vi "Request Parse.vi"(11 "WSGI Request":T2) -> (3 "Request":T1)   [LabVIEW 2021, in "HttpServer.lvlib"]
uses:
  HttpServer.lvlib
  TypeDefs/WSGI.ctl
  TypeDefs/Request.ctl
  <vilib>/Utility/miscctls.llb/LVMapReplaceAction.ctl
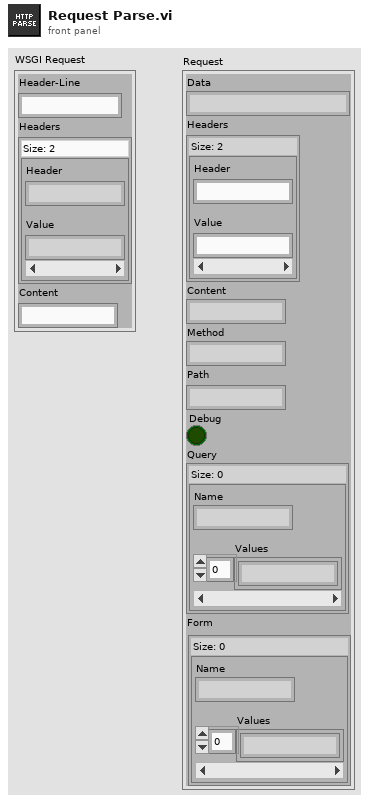
[diagram p1: front panel]
types:
  T1 = typedef "HttpServer.lvlib/Request.ctl" = cluster{"Data":string, "Headers":map{string, string}, "Content":string, "Method":string, "Path":string, "Debug":bool, "Query":map{string, string[]}, "Form":map{string, string[]}}
  T2 = typedef "HttpServer.lvlib/WSGI.ctl" = cluster{"Header-Line":string, "Headers":map{string, string}, "Content":string}
  T3 = typedef "LVMapReplaceAction.ctl" = enum32{"Modify Entry only if found", "Add or Modify Entry", "Delete Entry"}
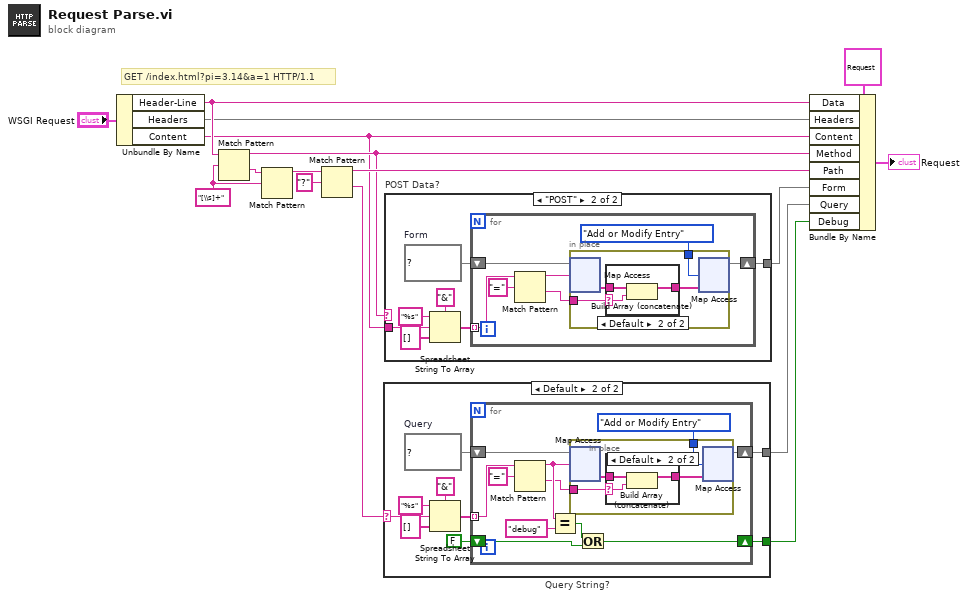
[diagram p0: block diagram]
diagram:
  w14 = "[\\s]+" ("regular expression")
  # "GET /index.html?pi=3.14&a=1 HTTP/1.1"
  n1 = Unbundle By Name("WSGI Request") -> ("Header-Line"=w11:string, "Headers"=w3:map{string, string}, "Content"=w2:string)
  n2 = Match Pattern(string=w11, regular expression=w14) -> (before substring=w4:string, after substring=w15:string)  [unwired: 1 in, 2 out]
  n3 = Match Pattern(string=w15, regular expression=w14) -> (before substring=w13:string)  [unwired: 1 in, 3 out]
  n4 = Match Pattern(string=w13, regular expression="?") -> (before substring=w10:string, after substring=w8:string)  [unwired: 1 in, 2 out]
  n5 = case "Query String?" shown="Default" w8 {
    selector: w8 -> [_ w22]
    tunnel: [_ w18] -> w6
    tunnel: [_ w17] -> w5
    frame "" {
    }
    frame Default {
      w20 = map{string, string[]} {}  # Query
      n6 = Spreadsheet String To Array(delimiter (Tab)="&", format string="%s", spreadsheet string=w22, array type (2D Dbl)=string[] []) -> (array=w21:string[])
      n7 = for {
        tunnel: w21 -> [w36] mode=indexing
        shift-right: [w27] -> w17
        shift-left: w20 -> [w30]
        shift-right: [w35] -> w18
        shift-left: FALSE -> [w34]
        n8 = Match Pattern(string=w36, regular expression="=") -> (before substring=w29:string, after substring=w28:string)  [unwired: 1 in, 2 out]
        n9 = Equal?(x=w29, y="debug" ("element")) -> (x = y?=w31:bool)
        n10 = in-place {
          in-place-border: w28 -> [w38]
          in-place-border: LVMapReplaceAction."Add or Modify Entry" ("action") -> [w40]
          n11 = in-place-map #1(w30, w29) -> (w39:string[])  [unwired: 1 in, 1 out]
          n12 = case shown="Default" w38 {
            selector: w38 -> [_ w42]
            tunnel: w39 -> [w41 w44]
            tunnel: [w41 w43] -> w37
            frame "" {
            }
            frame Default {
              n13 = Build Array (concatenate)(w44, w42) -> (w43:string[])
            }
          }
          n14 = in-place-map #1(w37, w40) -> (w27:map{string, string[]})  [unwired: 2 out]
        }
        n15 = Or(x=w31, y=w34) -> (x .or. y?=w35:bool)
      }
    }
  }
  n16 = case "POST Data?" shown="\"POST\"" w4 {
    tunnel: [_ w46] -> w1
    tunnel: w2 -> [_ w45]
    frame Default {
    }
    frame "POST" {
      w47 = map{string, string[]} {}  # Form
      n17 = Spreadsheet String To Array(delimiter (Tab)="&", format string="%s", spreadsheet string=w45, array type (2D Dbl)=string[] []) -> (array=w48:string[])
      n18 = for {
        tunnel: w48 -> [w58] mode=indexing
        shift-right: [w53] -> w46
        shift-left: w47 -> [w56]
        n19 = Match Pattern(string=w58, regular expression="=") -> (before substring=w55:string, after substring=w54:string)  [unwired: 1 in, 2 out]
        n20 = in-place {
          in-place-border: w54 -> [w60]
          in-place-border: LVMapReplaceAction."Add or Modify Entry" ("action") -> [w59]
          n21 = in-place-map #2(w56, w55) -> (w62:string[])  [unwired: 1 in, 1 out]
          n22 = case shown="Default" w60 {
            selector: w60 -> [_ w64]
            tunnel: w62 -> [w63 w66]
            tunnel: [w63 w65] -> w61
            frame "" {
            }
            frame Default {
              n23 = Build Array (concatenate)(w66, w64) -> (w65:string[])
            }
          }
          n24 = in-place-map #2(w61, w59) -> (w53:map{string, string[]})  [unwired: 2 out]
        }
      }
    }
  }
  n25 = Bundle By Name(cluster=T1 {"Data"="", "Headers"={}, "Content"="", "Method"="", "Path"="", "Debug"=FALSE, "Query"={}, "Form"={}} ("Request"), "Data"=w11, "Headers"=w3, "Content"=w2, "Method"=w4, "Path"=w10, "Form"=w1, "Query"=w5, "Debug"=w6) -> (→"Request":T1)
